vi "Periodic Tasks.vi"(8 "error in":errorcluster) -> ()   [LabVIEW 2015]
doc: "This VI runs in parallel to other tasks. It can contain as many user-defined periodic loops as you need. These can carry out PID or other sorts of timed response."
uses:
  <vilib>/Rock Robotics/WPI/Utilities/WPI_GetSetVariantRefNum.vi
  <vilib>/Rock Robotics/SystemInterfaces/Utilities/FPGA_UtilitiesRead LocalTime.vi
  <vilib>/Rock Robotics/Network Tables/NT Write Number.vi
  <vilib>/Rock Robotics/Network Tables/NT Write Numeric Array.vi
  ADI MXP IMU/ADI MXP IMU/FRC ADI MXP IMU.lvlib
panel:
  out "All PDP Currents":dbl[](array[numeric])
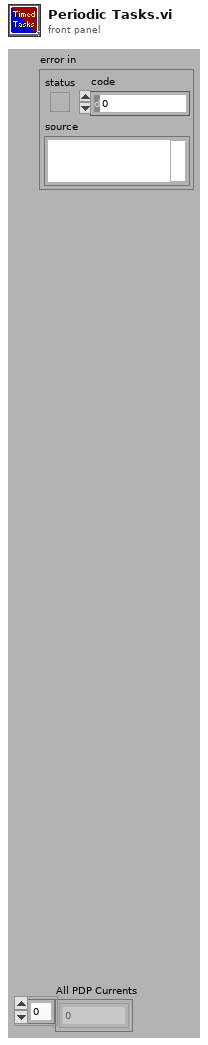
[diagram p1: front panel]
types:
  T1 = typedef "WPI_EncoderDevRef.ctl" = cluster{"DevStatus":errorcluster, "EncoderIndex":T2, "CounterIndex":T3, "DistancePerCount":dbl, "Decoding Type":T4}
  T2 = typedef "FPGA_EncoderIdx.ctl" = enum8{"Enc 0", "Enc 1", "Enc 2", "Enc 3", "Enc 4", "Enc 5", "Enc 6", "Enc 7", "Invalid"}
  T3 = typedef "FPGA_CounterCtrSystemIndex.ctl" = enum8{"Ctr 0", "Ctr 1", "Ctr 2", "Ctr 3", "Ctr 4", "Ctr 5", "Ctr 6", "Ctr 7", "Invalid"}
  T4 = typedef "WPI_EncoderType.ctl" = enum16{"1x", "2x", "4x"}
  T5 = typedef "FRC ADI MXP IMU.lvlib/WPI_AnalogDevicesIMUInterruptDevRef.ctl" = cluster{"SimpleGyroDevRef":T6, "InterruptRef":T8}
  T6 = typedef "FRC ADI MXP IMU.lvlib/WPI_AnalogDevicesIMUDevRef.ctl" = cluster{"DevStatus":errorcluster, "Handle":i32, "SPI Bus":T7, "Device Found":bool, "Sample Rate":dbl, "Device Ready":bool, "Yaw Axis":enum16{"X", "Y", "Z"}, "AHRS Algorithm":enum16{"Complementary", "Madgwick"}}
  T7 = typedef "spi_bus.ctl" = enum16{"SPI On-Board, CS0", "SPI On-Board, CS1", "SPI On-Board, CS2", "SPI On-Board, CS3", "SPI MXP", "Invalid"}
  T8 = typedef "WPI_InterruptRef.ctl" = cluster{"DevStatus":errorcluster, "InterruptIndex":T9}
  T9 = typedef "FPGA_InterruptIndex.ctl" = enum8{"0", "1", "2", "3", "4", "5", "6", "7", "Invalid"}
  T10 = typedef "WPI_JoystickDevRef.ctl" = cluster{"Device":T11}
  T11 = typedef "WPI_JoystickDeviceEnum.ctl" = enum16{"USB 0", "USB 1", "USB 2", "USB 3", "USB 4", "USB 5"}
  T12 = typedef "WPI_CompressorDevRef.ctl" = cluster{"DevStatus":errorcluster, "Pneumatics Control Module":u8}
  T13 = cluster{"X Angle":dbl, "Y Angle":dbl, "Z Angle":dbl}
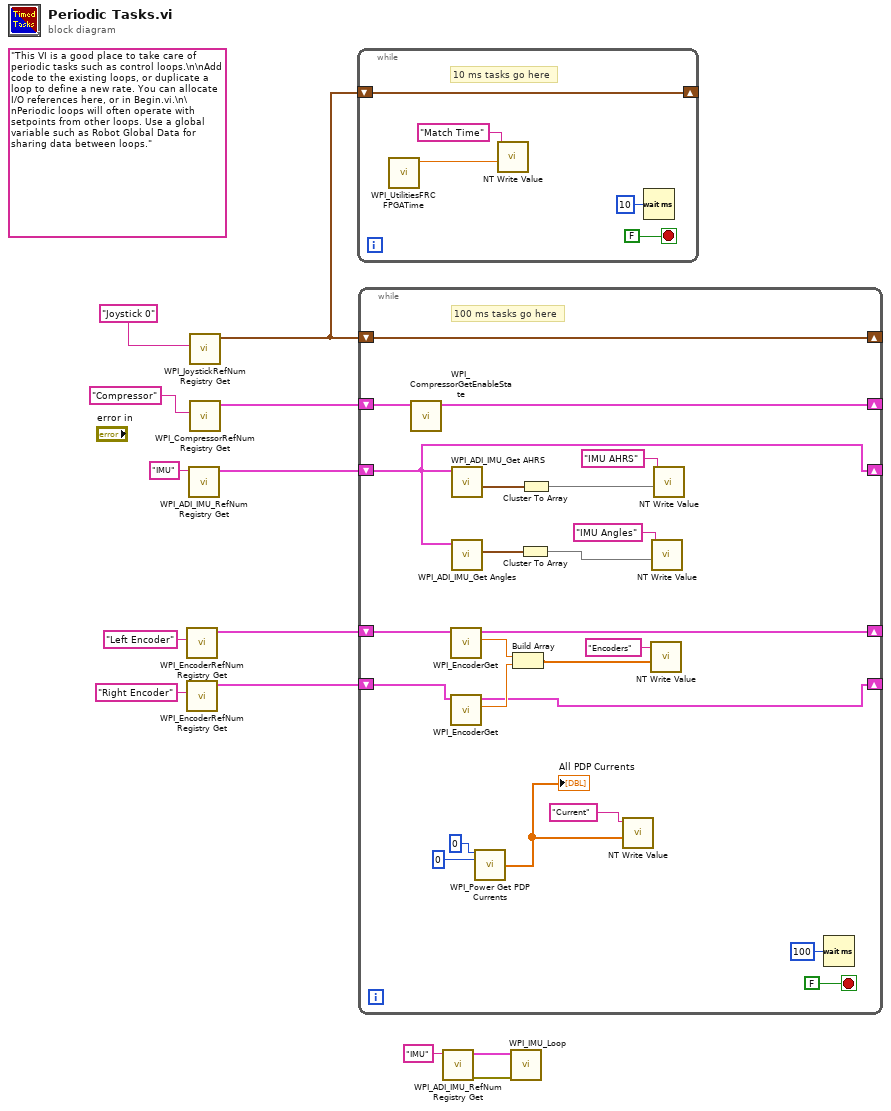
[diagram p0: block diagram]
diagram:
  (unwired) "This VI is a good place to take care of periodic tasks such as control loops.\n\nAdd code to the existing loops, or duplicate a loop to define a new rate. You can allocate I/O references here, or in Begin.vi.\n\nPeriodic loops will often operate with setpoints from other loops. Use a global variable such as Robot Global Data for sharing data between loops."
  n1 = call <vilib>:"WPI_EncoderRefNum Registry Get.vi"("refnum name"="Left Encoder") -> ("EncoderDevRef"=w2:T1)  [unwired: 9 in, 1 out]
  n2 = call <vilib>:"WPI_EncoderRefNum Registry Get.vi"("refnum name"="Right Encoder") -> ("EncoderDevRef"=w1:T1)  [unwired: 9 in, 1 out]
  n3 = call "WPI_ADI_IMU_RefNum Registry Get.vi"("refnum name"="IMU") -> ("ADI IMU Interrupt DevRef"=w5:T5)  [unwired: 9 in, 1 out]
  n4 = call <vilib>:"WPI_JoystickRefNum Registry Get.vi"("refnum name"="Joystick 0") -> ("JoystickDevRef"=w12:T10)  [unwired: 1 in, 9 out]
  n5 = call <vilib>:"WPI_CompressorRefNum Registry Get.vi"("refnum name"="Compressor") -> ("CompressorDevRef"=w10:T12)  [unwired: 9 in, 1 out]
  n6 = while {
    shift-right: [w16] -> _
    shift-left: w12 -> [w16]
    stop <- FALSE stop-if-true
    # "10 ms tasks go here"
    n7 = call <vilib>:"WPI_UtilitiesFRC FPGATime.vi"() -> ("FPGA Time"=w14:dbl)  [unwired: 10 in, 1 out]
    n8 = call-poly <vilib>:"NT Write Value.vi"("Numeric"=w14, "Name"="Match Time") -> ()  [unwired: 9 in, 1 out]
    n9 = Wait (ms)(milliseconds to wait=u32 10) -> ()  [unwired: 1 out]
  }
  n10 = while {
    shift-right: [w40] -> _
    shift-left: w12 -> [w40]
    shift-right: [w38] -> _
    shift-left: w10 -> [w39]
    shift-right: [w31] -> _
    shift-left: w5 -> [w31]
    shift-right: [w24] -> _
    shift-left: w2 -> [w26]
    shift-right: [w23] -> _
    shift-left: w1 -> [w25]
    stop <- FALSE stop-if-true
    # "100 ms tasks go here"
    n11 = call <vilib>:"WPI_CompressorGetEnableState.vi"("CompressorDevRef"=w39) -> ("CompressorDevRef"=w38:T12)  [unwired: 7 in, 3 out]
    n12 = call <vilib>:"WPI_EncoderGet.vi"("EncoderDevRef"=w26) -> ("Distance"=w29:dbl, "EncoderDevRef"=w24:T1)  [unwired: 5 in, 4 out]
    n13 = call <vilib>:"WPI_EncoderGet.vi"("EncoderDevRef"=w25) -> ("Distance"=w28:dbl, "EncoderDevRef"=w23:T1)  [unwired: 5 in, 4 out]
    n14 = call "WPI_ADI_IMU_Get AHRS.vi"("ADI IMU Interrupt DevRef"=w31) -> ("IMU AHRS DELTA"=w35:cluster{"Pitch":dbl, "Roll":dbl, "Yaw":dbl})  [unwired: 6 in, 4 out]
    n15 = call "WPI_ADI_IMU_Get Angles.vi"("ADI IMU Interrupt DevRef"=w31) -> ("IMU Angles"=w37:T13)  [unwired: 7 in, 3 out]
    n16 = call <vilib>:"WPI_Power Get PDP Currents.vi"("Power Distribution Panel (0)"=u8 0, "PDP Channel"=0) -> ("all currents (A)"=w20:dbl[])  [unwired: 11 in, 2 out]
    "All PDP Currents" <- w20
    n17 = Build Array(w29, w28) -> (w27:dbl[])
    n18 = Cluster To Array(cluster=w37) -> (array=w36:dbl[])
    n19 = Cluster To Array(cluster=w35) -> (array=w34:dbl[])
    n20 = call-poly <vilib>:"NT Write Value.vi"("Numeric Array"=w20, "Name"="Current") -> ()  [unwired: 9 in, 1 out]
    n21 = call-poly <vilib>:"NT Write Value.vi"("Numeric Array"=w27, "Name"="Encoders") -> ()  [unwired: 9 in, 1 out]
    n22 = call-poly <vilib>:"NT Write Value.vi"("Numeric Array"=w36, "Name"="IMU Angles") -> ()  [unwired: 9 in, 1 out]
    n23 = call-poly <vilib>:"NT Write Value.vi"("Numeric Array"=w34, "Name"="IMU AHRS") -> ()  [unwired: 9 in, 1 out]
    n24 = Wait (ms)(milliseconds to wait=u32 100) -> ()  [unwired: 1 out]
  }
  n25 = call "WPI_ADI_IMU_RefNum Registry Get.vi"("refnum name"="IMU") -> ("error out"=w8:errorcluster, "ADI IMU Interrupt DevRef"=w9:T5)  [unwired: 9 in]
  n26 = call "WPI_IMU_Loop.vi"("error in"=w8, "ADI IMU Interrupt DevRef"=w9) -> ()  [unwired: 8 in, 2 out]
